vi "Update tsettings from default_Core.vi"(6 "cRIO System Settings Cluster IN 2":T1={"CONFIG Folder - Relative Path "=path "Config", "FIFO Depth (# of elements)"=500000, "Avoid ALARM/ TRIP in transient regimes?"=TRUE, "Sample Rate [Hz]"=2048.0, "Processing interval [s]"=1.0, "Total number of channels to read from FPGA  (auto-calculated)"=0, "# of data to read-DMA (auto-calculated)"=0, "SysLog Interval (s)"=1, "Running Log Folder - Relative Path "=path "Logs/Running_Log", "Reset Log File - Relative Path "=path "Logs/ResetLog/cRIO_reset.txt", "Error Log File - Relative Path "=path "Logs/ErrLog/Errlogs.txt", "Ring Buffer Size (# Log File Elements)"=86400, "CPU Usage Exceed Limit ()"=98.0, "CPU Usage Exceed Limit Delay (# of iterrations)"=60, "Free Memory Min Avail.  (%)"=15.0, "Base CoDiS Folder"=path "c/CoDiS", "Archive Log Folder - Relative Path "=path "Logs/Archive_Logs", "Avail. Drive Space Limit to do Archive (%)"=20.0, "Mediator IP address"="10.50.10.2", "Mediator Communication TCP/IP Port"=2059, "Used channels (from FPGA) per units -Auto calculated"=[], "# DMA FIFO Fulls File - Relative Path "=path "Logs/ResetLog/Number of DMA FIFO Fulls.txt", "Log Status Parameters in cRIO Ring Buffer"=TRUE, "Channels Input Configuration (has to be defined for all available AI)"=[], "Index to check OL and SC (from FPGA) per units and channels -Auto calculated)"=[], "System not OK? (Auto-calculated)"=FALSE, "System not OK Relay Number (-1 = none, 0,..., MAX)"=-1, "Use normal (T) or inverse (F) relay logic for given relay (size of array equals to number of relays)?"=[], "U32 Relay Output (Auto-calculated)"=0, "cRIO Source"=enum."Not Used", "Check DMA FIFO Full?"=FALSE, "Modbus Settings"={"Modbus Communication Port"=502, "Run as Modbus Server/Slave? (FALSE=Modbus Client/Master)"=TRUE, "Modbus Slave Remote IP Address (if Run as Modbus Server/Slave?=FALSE)"=""}, "Time Synchronization Settings"={"Enable Time Synchronization"=FALSE, "Time Server IP Address (if Enable Time Synchronization=TRUE)"=""}} {"Channels Input Configuration (has to be defined for all available AI)" items=["AC Coupled", "DC Coupled", "IEPE AC Coupled", "Not DSA Channel"]}, 8 "cRIO System Settings Cluster IN":T1={"CONFIG Folder - Relative Path "=path "Config", "FIFO Depth (# of elements)"=500000, "Avoid ALARM/ TRIP in transient regimes?"=TRUE, "Sample Rate [Hz]"=2048.0, "Processing interval [s]"=1.0, "Total number of channels to read from FPGA  (auto-calculated)"=0, "# of data to read-DMA (auto-calculated)"=0, "SysLog Interval (s)"=1, "Running Log Folder - Relative Path "=path "Logs/Running_Log", "Reset Log File - Relative Path "=path "Logs/ResetLog/cRIO_reset.txt", "Error Log File - Relative Path "=path "Logs/ErrLog/Errlogs.txt", "Ring Buffer Size (# Log File Elements)"=86400, "CPU Usage Exceed Limit ()"=98.0, "CPU Usage Exceed Limit Delay (# of iterrations)"=60, "Free Memory Min Avail.  (%)"=15.0, "Base CoDiS Folder"=path "c/CoDiS", "Archive Log Folder - Relative Path "=path "Logs/Archive_Logs", "Avail. Drive Space Limit to do Archive (%)"=20.0, "Mediator IP address"="10.50.10.2", "Mediator Communication TCP/IP Port"=2059, "Used channels (from FPGA) per units -Auto calculated"=[], "# DMA FIFO Fulls File - Relative Path "=path "Logs/ResetLog/Number of DMA FIFO Fulls.txt", "Log Status Parameters in cRIO Ring Buffer"=TRUE, "Channels Input Configuration (has to be defined for all available AI)"=[3, 3, 3, 3, 3, 3, 3, 3, 3, 3, 3, 3, 3, 3, 3, 3, 3, 3, 3, 3, 3, 3, 3, 3, 3, 3, 3, 3, 3, 3, 3, 3, 3, 3, 3, 3, 3, 3, 3, 3, 3, 3, 3, 3, 3, 3, 3, 3, 2, 2, 2, 2, 2, 2, 2, 2, 2, 2, 2, 2], "Index to check OL and SC (from FPGA) per units and channels -Auto calculated)"=[], "System not OK? (Auto-calculated)"=FALSE, "System not OK Relay Number (-1 = none, 0,..., MAX)"=-1, "Use normal (T) or inverse (F) relay logic for given relay (size of array equals to number of relays)?"=[TRUE, TRUE, TRUE, TRUE, TRUE, TRUE, TRUE, TRUE], "U32 Relay Output (Auto-calculated)"=0, "cRIO Source"=enum."Source 1", "Check DMA FIFO Full?"=FALSE, "Modbus Settings"={"Modbus Communication Port"=502, "Run as Modbus Server/Slave? (FALSE=Modbus Client/Master)"=TRUE, "Modbus Slave Remote IP Address (if Run as Modbus Server/Slave?=FALSE)"=""}, "Time Synchronization Settings"={"Enable Time Synchronization"=FALSE, "Time Server IP Address (if Enable Time Synchronization=TRUE)"=""}} {"Channels Input Configuration (has to be defined for all available AI)" items=["AC Coupled", "DC Coupled", "IEPE AC Coupled", "Not DSA Channel"]}, 9 "1D array of Pan Cluster IN":T12[](array[typedef]) {"Absolute Minimum Air Gap per Plane"."Absolute AG Minimum Pole Number" format="%.3f"; "Absolute Minimum Air Gap per Plane"."Absolute AG Minimum Value" format="%.3f"; "Magnetic Field Data"."Maximum by Pole Number" format="%.3f"; "Air Gap Data"."Minimum by Pole Number" format="%.3f"; "Orbit(s) - XY"."Orbit XY Graphs (Synthesized from Selected Harmonics and DC)"."?" format="%.3f"; "Orbit(s) - XY"."Orbit XY Graphs (Synthesized from Selected Harmonics and DC)"."?" format="%.3f"; "Orbit(s) - XY"."Orbit XY Graphs (Glided and Averaged on One Revolution)"."?" format="%.3f"; "Orbit(s) - XY"."Orbit XY Graphs (Glided and Averaged on One Revolution)"."?" format="%.3f"; "Orbit(s) - XY"."Orbit XY Graphs (Unaveraged)"."?" format="%.3f"; "Orbit(s) - XY"."Orbit XY Graphs (Unaveraged)"."?" format="%.3f"}, 10 "1D array of Waveform Cluster IN":T6[](array[typedef]) {"Analysis Parameters"."SP2Pmax"."Filter Parameters"."low cutoff freq: fl" format="%0.4f"; "Analysis Parameters"."SP2Pmax"."Filter Parameters"."high cutoff freq: fh" format="%0.2f"; "Analysis Parameters"."LoadAngleDelta"."Multiplication Factor" format="%.1f"; "Analysis Parameters"."LoadAngleDelta"."What harmonic? (for example 24th (48 pole machine))" format="%.1f"; "Analysis Parameters"."Peak2Peak"."Filter Parameters"."low cutoff freq: fl" format="%0.4f"; "Analysis Parameters"."Peak2Peak"."Filter Parameters"."high cutoff freq: fh" format="%0.2f"; "Analysis Parameters"."RMS"."Filter Parameters"."order" format="%0.4f"; "Analysis Parameters"."RMS"."Filter Parameters"."low cutoff freq: fl" format="%0.2f"; "Analysis Parameters"."RMS"."Filter Parameters"."high cutoff freq: fh" format="%0.2f"; "Analysis Parameters"."EqPeak"."Filter Parameters"."low cutoff freq: fl" format="%0.4f"; "Analysis Parameters"."EqPeak"."Filter Parameters"."high cutoff freq: fh" format="%0.2f"; "Analysis Parameters"."Peak"."Filter Parameters"."low cutoff freq: fl" format="%0.4f"; "Analysis Parameters"."Peak"."Filter Parameters"."high cutoff freq: fh" format="%0.2f"; "Analysis Parameters"."snPh"."What harmonic?" format="%.1f"; "Analysis Parameters"."snA"."Multiplication Factor" format="%.1f"; "Analysis Parameters"."snA"."What harmonic?" format="%.1f"; "Analysis Parameters"."Smax"."Filter Parameters"."low cutoff freq: fl" format="%0.4f"; "Analysis Parameters"."Smax"."Filter Parameters"."high cutoff freq: fh" format="%0.2f"; "Analysis Parameters"."RPM"."Signal Threshold" format="%.1f"}, 11 "System_settings IN":T4={"Units in the system"=[], "dBase names by units"=[], "TCP/IP processing units addresses"=[], "TCP/IP server address"="", "dBase User Name_Cli"="codis_cli", "dBase User Password_Cli"="codis_cli", "dBase User Name_Med"="codis_med_wrt", "dBase User Password_Med"="codis_med_wrt", "Sampling rate [Hz]"=0.0, "FTP Server User name, cRIO"="", "FTP Server Password, cRIO"="", "OnScreenKeyboardPopUp"=FALSE, "Number of points to collect"=0, "Main Window has title bar?"=FALSE, "Demo?"=FALSE, "dBase - Limit # of  elements to read"=0, "dBase Backup"={"dBase Backup Base Folder"="c:\\codis\\backup\\", "Remote dBase Backup Configured?"=TRUE}, "System Status"={"System Monitor Refresh Rate (ms)"=10000, "System Status Log  File"="c:\\codis\\system_info.txt", "Max number of elements to read\n"=26611200}, "Number of points to average for stationary state"=[60], "Number of points to collect for saving waveforms per channel"=[60], "Sources per Unit"=[], "TCP/IP_client_mediator_communication ports"=2058, "TCP/IP processing_units _mediator_communication ports"=2055}) -> ()   [LabVIEW 2014]
uses:
  common/typedefs/Pan_Cluster_Core.ctl
  common/typedefs/Condition_Vector_Cluster_Core.ctl
  common/typedefs/Unit_Names_Core.ctl
  common/typedefs/Data_Sources_Core.ctl
  common/typedefs/Waveforms_Cluster_Core.ctl
  common/typedefs/Types_of_Signals_Core.ctl
  common/typedefs/Types_of_Analyses_Core.ctl
  common/typedefs/Analysis_Parameters_Cluster_Core.ctl
  <vilib>/Analysis/3filter.llb/Filter Passband Type.ctl
  common/typedefs/Integration_Types_Core.ctl
  common/typedefs/System_Settings_Cluster_Client_Mediator_Core.ctl
  common/typedefs/cRIO_System_Settings_Cluster_Core.ctl
  common/typedefs/DSA_Channels_Configuration_Core.ctl
  common/typedefs/dBase_Tables_Core.ctl
  common/typedefs/tsettings_Core.ctl
  <vilib>/addons/database/Connection.llb/DB Tools Open Connec (String).vi
  <vilib>/addons/database/NI_Database_API.lvlib
  <vilib>/Analysis/NI_AALBase.lvlib
panel:
  out "error out":errorcluster
  out "file error":errorcluster
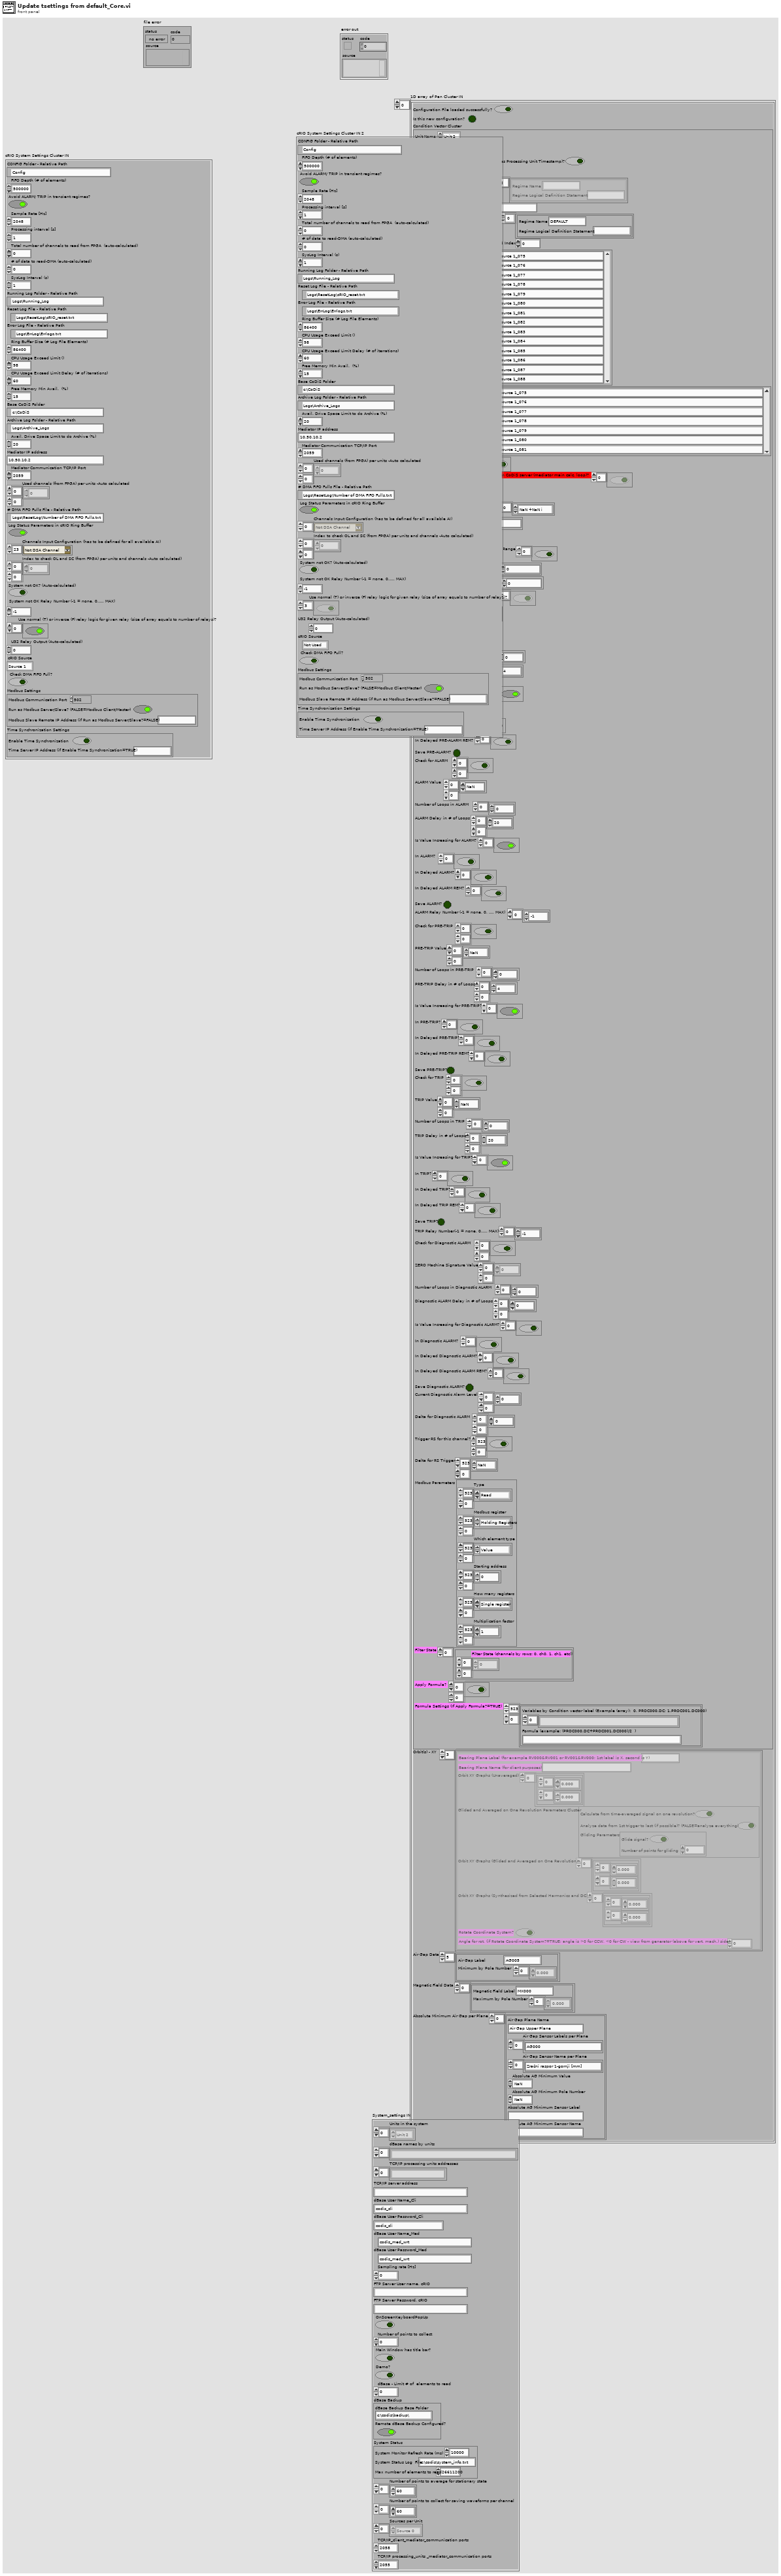
[diagram p1: front panel]
types:
  T1 = typedef "cRIO_System_Settings_Cluster_Core.ctl" = cluster{"CONFIG Folder - Relative Path ":path, "FIFO Depth (# of elements)":u32, "Avoid ALARM/ TRIP in transient regimes?":bool, "Sample Rate [Hz]":sgl, "Processing interval [s]":sgl, "Total number of channels to read from FPGA  (auto-calculated)":u32, "# of data to read-DMA (auto-calculated)":u32, "SysLog Interval (s)":u32, "Running Log Folder - Relative Path ":path, "Reset Log File - Relative Path ":path, "Error Log File - Relative Path ":path, "Ring Buffer Size (# Log File Elements)":u32, "CPU Usage Exceed Limit ()":sgl, "CPU Usage Exceed Limit Delay (# of iterrations)":u32, "Free Memory Min Avail.  (%)":sgl, "Base CoDiS Folder":path, "Archive Log Folder - Relative Path ":path, "Avail. Drive Space Limit to do Archive (%)":sgl, "Mediator IP address":string, "Mediator Communication TCP/IP Port":u16, "Used channels (from FPGA) per units -Auto calculated":i32[][], "# DMA FIFO Fulls File - Relative Path ":path, "Log Status Parameters in cRIO Ring Buffer":bool, "Channels Input Configuration (has to be defined for all available AI)":T2[], "Index to check OL and SC (from FPGA) per units and channels -Auto calculated)":i32[][], "System not OK? (Auto-calculated)":bool, "System not OK Relay Number (-1 = none, 0,..., MAX)":i16, "Use normal (T) or inverse (F) relay logic for given relay (size of array equals to number of relays)?":bool[], "U32 Relay Output (Auto-calculated)":u32, "cRIO Source":T3, "Check DMA FIFO Full?":bool, "Modbus Settings":cluster{"Modbus Communication Port":u16, "Run as Modbus Server/Slave? (FALSE=Modbus Client/Master)":bool, "Modbus Slave Remote IP Address (if Run as Modbus Server/Slave?=FALSE)":string}, "Time Synchronization Settings":cluster{"Enable Time Synchronization":bool, "Time Server IP Address (if Enable Time Synchronization=TRUE)":string}}
  T2 = typedef "DSA_Channels_Configuration_Core.ctl" = u16
  T3 = typedef "Data_Sources_Core.ctl" = enum16{"Not Used", "Source 0", "Source 1", "Source 2", "Source 3", "Source 4", "Source 5", "Source 6", "Source 7", "Source 8", "Source 9", "Source 10", "Source 11", "Source 12", "Source 13", "Source 14", "Source 15", "Source 16", "Source 17", "Source 18", "Source 19", "Source 20"}
  T4 = typedef "System_Settings_Cluster_Client_Mediator_Core.ctl" = cluster{"Units in the system":T5[], "dBase names by units":string[], "TCP/IP processing units addresses":string[], "TCP/IP server address":string, "dBase User Name_Cli":string, "dBase User Password_Cli":string, "dBase User Name_Med":string, "dBase User Password_Med":string, "Sampling rate [Hz]":dbl, "FTP Server User name, cRIO":string, "FTP Server Password, cRIO":string, "OnScreenKeyboardPopUp":bool, "Number of points to collect":u32, "Main Window has title bar?":bool, "Demo?":bool, "dBase - Limit # of  elements to read":u32, "dBase Backup":cluster{"dBase Backup Base Folder":string, "Remote dBase Backup Configured?":bool}, "System Status":cluster{"System Monitor Refresh Rate (ms)":u32, "System Status Log  File":string, "Max number of elements to read\n":i64}, "Number of points to average for stationary state":i32[], "Number of points to collect for saving waveforms per channel":i32[], "Sources per Unit":T3[], "TCP/IP_client_mediator_communication ports":u16, "TCP/IP processing_units _mediator_communication ports":u16}
  T5 = typedef "Unit_Names_Core.ctl" = enum16{"Not used", "Unit 1", "Unit 2", "Unit 3", "Unit 4", "Unit 5", "Unit 6", "Unit 7", "Unit 8", "Unit 9"}
  T6 = typedef "Waveforms_Cluster_Core.ctl" = cluster{"Configuration File loaded successfully? ":bool, "Is this new configuration?":bool, "Unit Name":T5, "Waveform Source":T3[], "Use CoDiS server Timestamp (on FALSE uses Processing Unit Timestamp)?":bool, "Sampling Rate [Hz]":u32[], "Timestamp (DBL)":dbl, "Mode of Operation - Normal":string, "Mode of Operation - Diagnostic":string, "Waveform Physical Channel":u16[], "Waveform Label":string[], "Waveform Name":string[], "Signal Type":cluster{"Signal Type":T7, "# of signal of particular type":u8}[], "Is this Main Trigger Signal?":bool[], "Slope":dbl[], "Intercept":dbl[], "Waveform Values":sgl[][], "Analyse?":bool[], "Save to database?":bool[], "Analyses to Perform":T8[][], "Perform this analysis on a CoDiS server?":bool[][], "General Parameters":cluster{"Number of Poles":u8, "Grid Frequency":sgl}, "Analysis Parameters":T9[][], "Save now to dBase?":bool, "Waveform Length for Saving [s]":u16, "Pretrigger Length when Saving Waveform [s]":u16, "Next Timestamp to autosave at (DBL)":dbl, "Description of Waveforms Events":string, "Event Type":string, "Save next RS event entirely? (on FALSE uses How many basic (acquisition) blocks of data (loops) to save?":bool, "Regime Name for which to save next RS event entirely":string, "Integration type":T11[], "Channel not OK?":bool[], "Channel Not OK?  Relay Number (-1 = none, 0, ..., MAX)":i16[], "Array of FPGA Filter Parameters":cluster{"Filter signal?":bool, "filter type":T10, "high cutoff freq: fh":dbl, "low cutoff freq: fl":dbl, "order":i32}[][], "Pre-Alarm Delay in Number of Loops ":u16, "Pre-Trip Delay in Number of Loops ":u16}
  T7 = typedef "Types_of_Signals_Core.ctl" = enum16{"Not Used", "Trigger (TRG???)", "Relative Vibrations (RV???)", "Absolute Vibrations (AV???)", "Air Gap (AG???)", "Magnetic Field (MX???)", "Voltage (VOL???)", "Current (CURR???)", "Process (PROC???)", "Cavitation (CAV???)", "Non Standard (NONST???)", "Axial Displacement (AXD???)", "Absolute Vibrations Stator Core (AVSC???)"}
  T8 = typedef "Types_of_Analyses_Core.ctl" = enum16{"Exit Analysis Loop", "Do Nothing", "RPM", "Smax", "SP2Pmax", "snA", "snPh", "Rest", "Peak", "EqPeak", "Peak2Peak", "RMS", "DC", "DC from Extrema", "Min Value", "Max Value", "Min Value by Pole", "Max Value by Pole", "Max Diff by Pole", "Max Diff Pole Number", "Min from Extrema", "Max from Extrema", "Active Power from DFT", "Active Power by Integration", "Reactive Power from DFT", "Reactive Power by Integration", "Apparent Power", "Ampl@Freq", "Phase Difference", "Load Angle Delta", "THD", "Signal Frequency", "Eta", "Non standard (CoDiS server - manual) 0", "Non standard (CoDiS server - manual) 1", "Non standard (CoDiS server - manual) 2", "Non standard (CoDiS server - manual) 3", "Non standard (CoDiS server - manual) 4", "Non standard (CoDiS server - manual) 5", "Non standard (CoDiS server - manual) 6", "Non standard (CoDiS server - manual) 7", "Non standard (CoDiS server - manual) 8", "Non standard (CoDiS server - manual) 9", "Non standard (CoDiS server - manual) 10", "Non standard (CoDiS server - manual) 11", "Non standard (CoDiS server - manual) 12", "Non standard (CoDiS server - manual) 13", "Non standard (CoDiS server - manual) 14", "Non standard (CoDiS server - manual) 15", "Non standard (CoDiS server - manual) 16", "Non standard (CoDiS server - manual) 17", "Non standard (CoDiS server - manual) 18", "Non standard (CoDiS server - manual) 19", "CosFi", "Total THD", "Crest Factor"}
  T9 = typedef "Analysis_Parameters_Cluster_Core.ctl" = cluster{"DC":cluster{"Analyze data from 1st trigger to last (if possible)? (FALSE=analyze everything)":bool}, "DCExtrema":cluster{"Calculate DC from all Pole Values":bool, "Poles to use in DC calculation (if Calculate DC from all Pole Values is FALSE)":u8[], "Condition Vector Label begin Part (MinPole or MaxPole)":string, "Addition to Condition Vector Label (example: 000)":string}, "RPM":cluster{"Signal Threshold":sgl, "Pulse Width (should be >= 2 depending on signal noise)":i32, "Trigger on rising edge? (FALSE=trigger on falling)":bool}, "Smax":cluster{"Combine with which Waveform Label? (for example: RV001)":string, "Calculate from time-averaged signal on one revolution?":bool, "Analyze data from 1st trigger to last (if possible)? (FALSE=analyze everything)":bool, "Filter Parameters":cluster{"Filter signal?":bool, "filter type":T10, "high cutoff freq: fh":dbl, "low cutoff freq: fl":dbl, "order":i32, "Process as ring-buffer signal?":bool}, "Gliding Parameters":cluster{"Glide signal?":bool, "Number of points for gliding":u16}, "Average all calculated values for Smax - if present (each revolution)? (FALSE=take absolute maximum)":bool, "Addition to Condition Vector Label (example: 000)":string}, "SP2Pmax":cluster{"Combine with which Waveform Label? (for example: RV001)":string, "Calculate from time-averaged signal on one revolution?":bool, "Analyze data from 1st trigger to last (if possible)? (FALSE=analyze everything)":bool, "Filter Parameters":cluster{"Filter signal?":bool, "filter type":T10, "high cutoff freq: fh":dbl, "low cutoff freq: fl":dbl, "order":i32, "Process as ring-buffer signal?":bool}, "Gliding Parameters":cluster{"Glide signal?":bool, "Number of points for gliding":u16}, "Average all calculated values for SP2Pmax - if present (each revolution)? (FALSE=take absolute maximum)":bool, "Addition to Condition Vector Label (example: 000)":string}, "snA":cluster{"What harmonic?":sgl, "Calculate Amplitude (TRUE) or RMS (FALSE)?":bool, "Multiplication Factor":sgl, "Calculate Amplitude for Air Gap type signals? (from MinPole Values)":bool}, "snPh":cluster{"What harmonic?":sgl}, "Peak":cluster{"Calculate from time-averaged signal (one-revolution)?":bool, "Analyze data from 1st trigger to last (if possible)? (FALSE=analyze everything)":bool, "Filter Parameters":cluster{"Filter signal?":bool, "filter type":T10, "high cutoff freq: fh":dbl, "low cutoff freq: fl":dbl, "order":i32, "Process as ring-buffer signal?":bool}, "Gliding Parameters":cluster{"Glide signal?":bool, "Number of points for gliding":u16}, "Average all calculated values for Peak - if present (each revolution)? (FALSE=take absolute maximum)":bool, "Addition to Condition Vector Label (example: 000)":string}, "Peak2Peak":cluster{"Calculate from time-averaged signal (one-revolution)?":bool, "Analyze data from 1st trigger to last (if possible)? (FALSE=analyze everything)":bool, "Gliding Parameters":cluster{"Glide signal?":bool, "Number of points for gliding":u16}, "Filter Parameters":cluster{"Filter signal?":bool, "filter type":T10, "high cutoff freq: fh":dbl, "low cutoff freq: fl":dbl, "order":i32, "Process as ring-buffer signal?":bool}, "Average all calculated values for Peak2Peak - if present (each revolution)? (FALSE=take absolute maximum)":bool, "Addition to Condition Vector Label (example: 000)":string}, "EqPeak":cluster{"Calculate from time-averaged signal (one-revolution)?":bool, "Analyze data from 1st trigger to last (if possible)? (FALSE=analyze everything)":bool, "Average all calculated values for EqPeak - if present (each revolution)? (FALSE=take absolute maximum)":bool, "Filter Parameters":cluster{"Filter signal?":bool, "filter type":T10, "high cutoff freq: fh":dbl, "low cutoff freq: fl":dbl, "order":i32, "Process as ring-buffer signal?":bool}, "Which Condition Vector Label addition to use for RMS (example: 001)":string, "Addition to Condition Vector Label (example: 000)":string}, "RMS":cluster{"Calculate from time-averaged signal (one-revolution)?":bool, "Analyze data from 1st trigger to last (if possible)? (FALSE=analyze everything)":bool, "Subtract DC before RMS calculation?":bool, "Filter Parameters":cluster{"Filter signal?":bool, "filter type":T10, "high cutoff freq: fh":dbl, "low cutoff freq: fl":dbl, "order":i32, "Process as ring-buffer signal?":bool}, "Gliding Parameters":cluster{"Glide signal?":bool, "Number of points for gliding":u16}, "Average all calculated values for RMS - if present (each revolution)? (FALSE=take absolute maximum)":bool, "Addition to Condition Vector Label (example: 000)":string}, "Rest":cluster{"Calculate from all calculated harmonics?":bool, "Condition Vector Label to use for substraction (if Calculate from all calculated harmonics?=FALSE)":string[], "Calculate by subtracting from EqPeak Value? (FALSE=calculate by subtracting from RMS Value)":bool, "Which Condition Vector Label addition to use for EqPeak (example: 001)":string, "Addition to Condition Vector Label (example: 000)":string}, "MinByPole":cluster{"First Pole Number after Trigger (indexes correspond to Normal regime settings)":u8[], "Are Pole Numbers in ascending order in time?  (indexes correspond to Normal regime settings)":bool[], "Average all calculated values for that Pole? (FALSE=take absolute minimum)":bool, "Coerce Upper Limit":sgl, "Compensate 1st harmonic in waveform?":bool}, "MinExtrema":cluster{"Calculate Min Extrema from all Pole Values":bool, "Poles to use in Min Extrema calculation (if Calculate Min Extrema from all Pole Values is FALSE)":u8[], "Condition Vector Label begin Part (MinPole or MaxPole)":string}, "MaxByPole":cluster{"First Pole Number after Trigger (indexes correspond to Normal regime settings)":u8[], "Are Pole Numbers in ascending order in time? (indexes correspond to Normal regime settings)":bool[], "Average all calculated values for that Pole? (FALSE=take absolute maximum)":bool, "Calculate with abs(Signal)?":bool, "Subtract DC before calculation?":bool, "Coerce Lower Limit":sgl}, "MaxExtrema":cluster{"Calculate Max Extrema from all Pole Values":bool, "Poles to use in Max Extrema calculation (if Calculate Max Extrema from all Pole Values is FALSE)":u8[], "Condition Vector Label begin Part (MinPole or MaxPole)":string}, "MaxDiffByPole":cluster{"First Pole Number after Trigger (indexes correspond to Normal regime settings)":u8[], "Are Pole Numbers in ascending order in time? (indexes correspond to Normal regime settings)":bool[], "Condition Vector Label begin Part (MinPole or MaxPole)":string}, "Min":cluster{"Analyze data from 1st trigger to last (if possible)? (FALSE=analyze everything)":bool, "Calculate from time-averaged signal on one revolution?":bool, "Gliding Parameters":cluster{"Glide signal?":bool, "Number of points for gliding":u16}, "Average all calculated values for Min - if present (each revolution)? (FALSE=take absolute maximum)":bool}, "Max":cluster{"Analyze data from 1st trigger to last (if possible)? (FALSE=analyze everything)":bool, "Calculate from time-averaged signal on one revolution?":bool, "Gliding Parameters":cluster{"Glide signal?":bool, "Number of points for gliding":u16}, "Average all calculated values for Max - if present (each revolution)? (FALSE=take absolute maximum)":bool}, "ActivePower":cluster{"Calculate from Phase Voltages and Currents?":bool, "Phase Voltage Condition Vector Label (R, S, T) (for example: VOL000.s24.00A, VOL001.s24.00A, VOL002.s24.00A)":string[], "Phase Current Condition Vector Label (R, S, T) (for example: CURR000.s24.00A, CURR001.s24.00A, CURR002.s24.00A)":string[]}, "ReactivePower":cluster{"Calculate from Phase Voltages and Currents?":bool, "Phase Voltage Condition Vector Label (R, S, T) (for example: VOL000.s24.00A, VOL001.s24.00A, VOL002.s24.00A)":string[], "Phase Current Condition Vector Label (R, S, T) (for example: CURR000.s24.00A, CURR001.s24.00A, CURR002.s24.00A)":string[]}, "LoadAngleDelta":cluster{"What harmonic? (for example 24th (48 pole machine))":sgl, "Delta0":sgl, "Which Voltage Waveform Label? (for example: VOL000)":string, "Combine (multiply) with which Air Gap Waveform Label? (for example: AG000)":string, "Multiplication Factor":sgl}, "ActivePowerByIntegration":cluster{"Phase Voltage Waveform Labels (R,S,T)":string[], "Phase Current Waveform Labels (R,S,T)":string[], "Analyze data from 1st trigger to last (if possible)? (FALSE=analyze everything)":bool}, "RectivePowerByIntegration":cluster{"Phase Voltage Waveform Vector Labels (R,S,T)":string[], "Phase Current Waveform Labels (R,S,T)":string[], "System Electric Frequency [Hz]":sgl, "Analyze data from 1st trigger to last (if possible)? (FALSE=analyze everything)":bool}, "Ampl@Freq":cluster{"Frequency [Hz]":sgl, "Calculate Amplitude? (FALSE=calculate RMS)":bool}, "PhaseDifference":cluster{"Combine with which Waveform Label?":string}, "CosFi":cluster{"Voltage Waveform Labels (R,S,T)":string[], "Current Waveform Labels (R,S,T)":string[]}, "Total THD":cluster{"THD Condition Vector Label (R, S, T) (for example: VOL000.THD, VOL001.THD, VOL002.THD)":string[]}, "Crest Factor":cluster{"Addition to Condition Vector Label (example: 000)":string, "Which Condition Vector Label addition to use for Peak (example: 001)":string, "Which Condition Vector Label addition to use for RMS (example: 001)":string}}
  T10 = typedef "NI_AALBase.lvlib/Filter Passband Type.ctl" = enum32{"Lowpass", "Highpass", "Bandpass", "Bandstop"}
  T11 = typedef "Integration_Types_Core.ctl" = enum16{"Do not integrate", "Integrate once", "Integrate twice"}
  T12 = typedef "Pan_Cluster_Core.ctl" = cluster{"Configuration File loaded successfully?":bool, "Is this new configuration?":bool, "Condition Vector Cluster":T13, "Orbit(s) - XY":cluster{"Bearing Plane Label (for example RV000&RV001 or RV001&RV000; 1st label is X, second is Y)":string, "Bearing Plane Name (for client purposes)":string, "Orbit XY Graphs (Unaveraged)":cluster{sgl[], sgl[]}[], "Glided and Averaged on One Revolution Parameters Cluster":cluster{"Calculate from time-averaged signal on one revolution?":bool, "Analyze data from 1st trigger to last (if possible)? (FALSE=analyze everything)":bool, "Gliding Parameters":cluster{"Glide signal?":bool, "Number of points for gliding":u16}}, "Orbit XY Graphs (Glided and Averaged on One Revolution)":cluster{sgl[], sgl[]}[], "Orbit XY Graphs (Synthesized from Selected Harmonics and DC)":cluster{sgl[], sgl[]}[], "Rotate Coordinate System?":bool, "Angle for rot. (if Rotate Coordinate System?=TRUE; angle is >0 for CCW, <0 for CW - view from generator (above for vert. mach.) side)":sgl}[], "Air Gap Data":cluster{"Air Gap Label":string, "Minimum by Pole Number":sgl[]}[], "Magnetic Field Data":cluster{"Magnetic Field Label":string, "Maximum by Pole Number":sgl[]}[], "Absolute Minimum Air Gap per Plane":cluster{"Air Gap Plane Name":string, "Air Gap Sensor Labels per Plane":string[], "Air Gap Sensor Name per Plane":string[], "Absolute AG Minimum Value":sgl, "Absolute AG Minimum Pole Number":sgl, "Absolute AG Minimum Sensor Label":string, "Absolute AG Minimum Sensor Name":string}[]}
  T13 = typedef "Condition_Vector_Cluster_Core.ctl" = cluster{"Unit Name":T5, "Source Name":T3[], "Use CoDiS server Timestamp (on FALSE uses Processing Unit Timestamp)?":bool, "Timestamp (DBL)":dbl, "Mode of Operation - Normal (Settings)":cluster{"Regime Name":string, "Regime Logical Definition Statement":string}[], "Mode of Operation - Normal":string, "Mode of Operation - Diagnostic (Settings)":cluster{"Regime Name":string, "Regime Logical Definition Statement":string}[], "Mode of Operation - Diagnostic Recognized Index":i16, "Condition Vector Label":string[], "Condition Vector Name":string[], "Is this Main Trigger Signal?":bool[], "Perform PRE-ALARM, ALARM, etc. Analysis on CoDiS server (mediator main calc. loop)?":bool[], "Trigger Indexes":u32[], "Condition Vector Values Complex (CDB)":cdb[], "Condition Vector Values":sgl[], "Save to dBase":bool[], "Check if Condition Vector Element is out of Range":bool[], "Condition Vector Low Limit Value":sgl[], "Condition Vector High Limit Value":sgl[], "Condition Vector Element out of Range":bool[], "Check for PRE-ALARM":bool[][], "PRE-ALARM Value":sgl[][], "Number of Loops in PRE-ALARM":u32[], "PRE-ALARM Delay in # of Loops":u16[][], "Is Value Increasing for PRE-ALARM?":bool[], "In PRE-ALARM?":bool[], "In Delayed PRE-ALARM?":bool[], "In Delayed PRE-ALARM REM?":bool[], "Save PRE-ALARM?":bool, "Check for ALARM":bool[][], "ALARM Value":sgl[][], "Number of Loops in ALARM":u32[], "ALARM Delay in # of Loops":u16[][], "Is Value Increasing for ALARM?":bool[], "In ALARM?":bool[], "In Delayed ALARM?":bool[], "In Delayed ALARM REM?":bool[], "Save ALARM?":bool, "ALARM Relay Number (-1 = none, 0, ..., MAX)":i16[], "Check for PRE-TRIP":bool[][], "PRE-TRIP Value":sgl[][], "Number of Loops in PRE-TRIP":u32[], "PRE-TRIP Delay in # of Loops":u16[][], "Is Value Increasing for PRE-TRIP?":bool[], "In PRE-TRIP?":bool[], "In Delayed PRE-TRIP?":bool[], "In Delayed PRE-TRIP REM?":bool[], "Save PRE-TRIP?":bool, "Check for TRIP":bool[][], "TRIP Value":sgl[][], "Number of Loops in TRIP":u32[], "TRIP Delay in # of Loops":u16[][], "Is Value Increasing for TRIP?":bool[], "In TRIP?":bool[], "In Delayed TRIP?":bool[], "In Delayed TRIP REM?":bool[], "Save TRIP?":bool, "TRIP Relay Number(-1 = none, 0,..., MAX)":i16[], "Check for Diagnostic ALARM":bool[][], "ZERO Machine Signature Value":dbl[][], "Number of Loops in Diagnostic ALARM":u32[], "Diagnostic ALARM Delay in # of Loops":u16[][], "Is Value Increasing for Diagnostic ALARM?":bool[], "In Diagnostic ALARM?":bool[], "In Delayed Diagnostic ALARM?":bool[], "In Delayed Diagnostic ALARM REM?":bool[], "Save Diagnostic ALARM?":bool, "Current Diagnostic Alarm Level":sgl[][], "Delta for Diagnostic ALARM":sgl[][], "Trigger RS for this channel?":bool[][], "Delta for RS Trigger":sgl[][], "Modbus Parameters":cluster{"Type":enum16{"Read", "Write", "None"}[][], "Modbus register":enum16{"Coils", "Discrete Inputs", "Input Registers", "Holding Registers"}[][], "Which element type":enum16{"Value", "Alarm", "Trip"}[][], "Starting address":u16[][], "How many registers":enum16{"Single register", "HI-LO", "LO-HI"}[][], "Multiplication factor":dbl[][]}, "Filter State":cluster{"Filter State (channels by rows: 0. ch0, 1. ch1, etc))":dbl[][]}[], "Apply Formula?":bool[][], "Formula Settings (If Apply Formula?=TRUE)":cluster{"Variables by Condition vector label (Example (array):  0. PROC000.DC; 1.PROC001.DC000)":string[], "Formula (example: (PROC000.DC+PROC001.DC000)/2  )":string}[][]}
  T14 = typedef "tsettings_Core.ctl" = enum16{"Waveform Cluster", "Pan Cluster", "Reference Waveform for AG RSS", "System Settings", "RunOut Vector"}
  T15 = typedef "dBase_Tables_Core.ctl" = string
  T16 = typedef "NI_Database_API.lvlib/Conn ObjectReference.ctl" = refnum<k1>
  T17 = cluster{"Number of records OUT":u64, "idUser":u64, "tSetting_TypeDef":T14, dbl, "Waveform Cluster DEFAULT":T6, "Administrator Cluster.Description":string, "Uploaded":u64}
  T18 = cluster{u64, "idUser":u64, i32, dbl, "cRIO System Settings Cluster IN 2":T1, "Administrator Cluster.Description":string, "Uploaded":u64}
  T19 = cluster{u64, "idUser":u64, "tSetting_TypeDef":T14, dbl, "Pan Cluster DEFAULT":T12, "Administrator Cluster.Description":string, "Uploaded":u64}
  T20 = cluster{u64, "idUser":u64, i32, dbl, "cRIO System Settings Cluster IN":T1, "Administrator Cluster.Description":string, "Uploaded":u64}
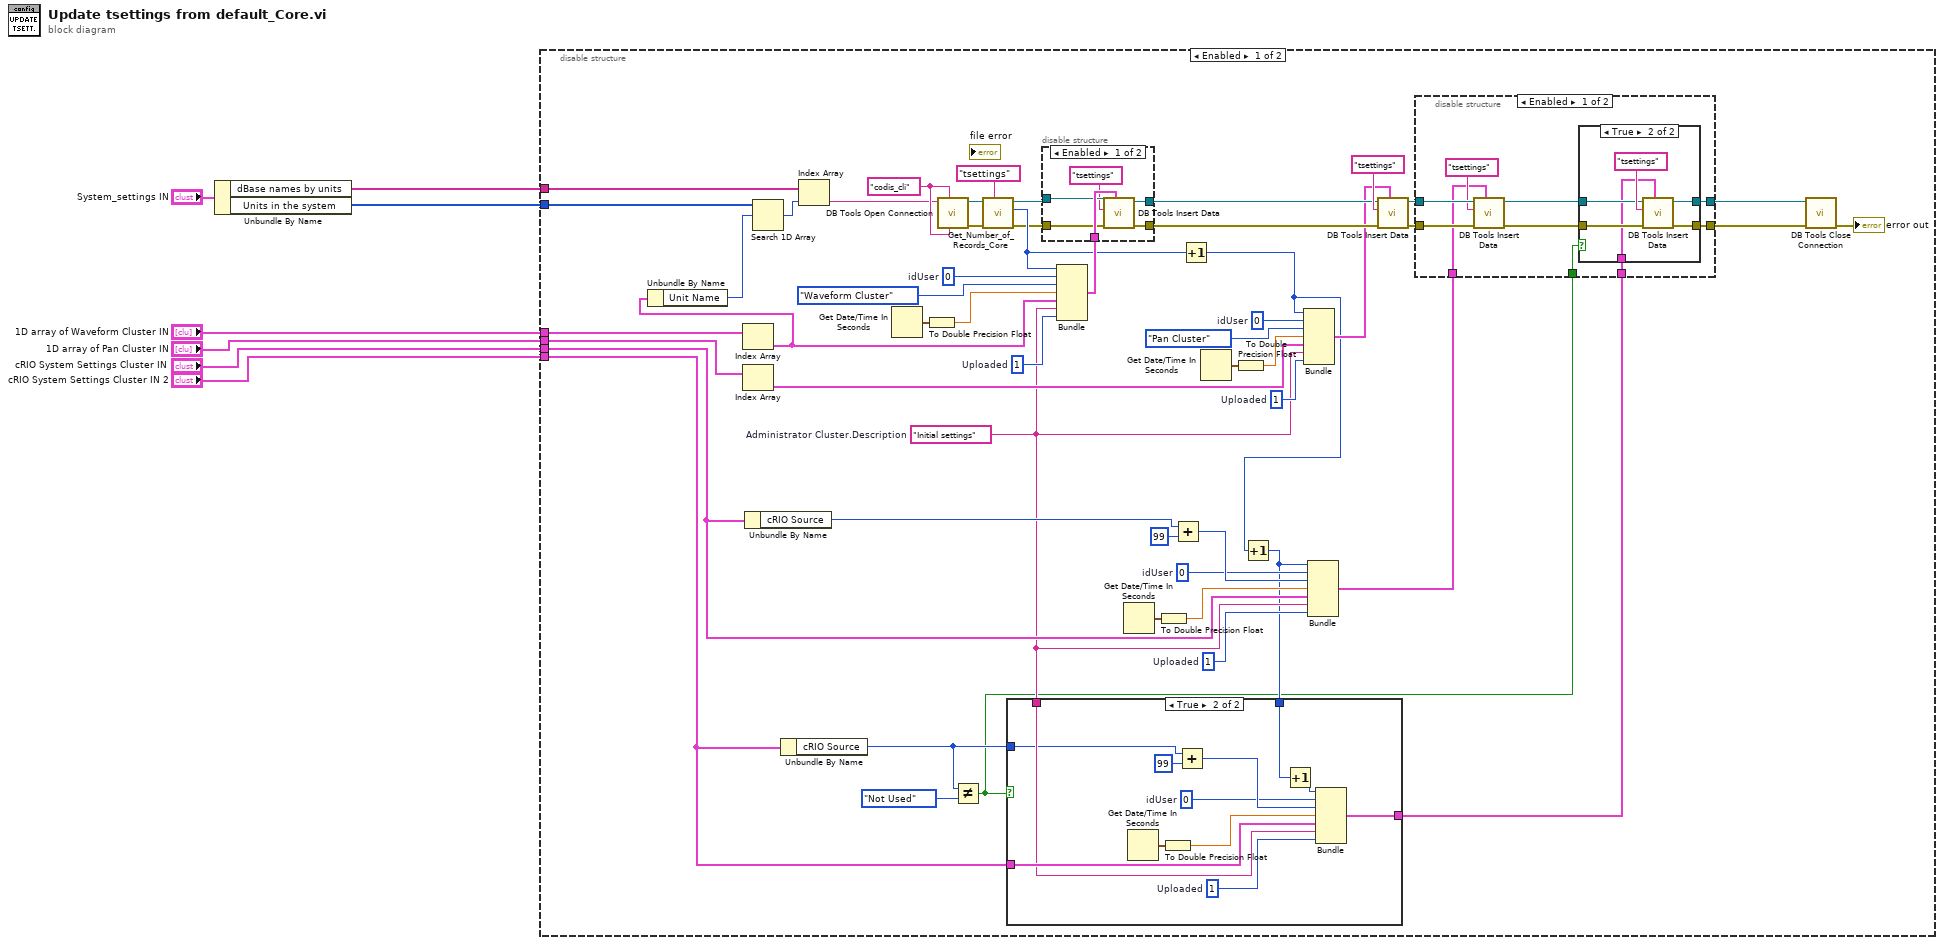
[diagram p0: block diagram]
diagram:
  n1 = Unbundle By Name("System_settings IN") -> ("dBase names by units"=w6:string[], "Units in the system"=w7:T5[])
  n2 = disable-structure shown="Enabled" {
    disable-tunnel: "1D array of Waveform Cluster IN" -> [w44 _]
    disable-tunnel: "1D array of Pan Cluster IN" -> [w43 _]
    disable-tunnel: "cRIO System Settings Cluster IN" -> [w34 _]
    disable-tunnel: "cRIO System Settings Cluster IN 2" -> [w30 _]
    disable-tunnel: w7 -> [w24 _]
    disable-tunnel: w6 -> [w21 _]
    frame Enabled {
      w41 = u64 1  # Uploaded
      w28 = u64 0  # idUser
      w29 = "Initial settings"  # Administrator Cluster.Description
      w52 = u64 1  # Uploaded
      w53 = u64 0  # idUser
      w55 = "codis_cli" ("password")
      w57 = u64 1  # Uploaded
      w58 = u64 0  # idUser
      n3 = Index Array(array=w44) -> (element=w23:T6)  [unwired: 1 in]
      n4 = Unbundle By Name(w23) -> ("Unit Name"=w22:T5)
      n5 = Index Array(array=w43) -> (element=w45:T12)  [unwired: 1 in]
      n6 = Unbundle By Name(w34) -> ("cRIO Source"=w33:T3)
      n7 = Search 1D Array(1D array=w24, element=w22) -> (index of element=w20:i32)  [unwired: 1 in]
      n8 = Unbundle By Name(w30) -> ("cRIO Source"=w17:T3)
      n9 = Index Array(array=w21, index=w20) -> (element=w19:string)
      n10 = Get Date/Time In Seconds() -> (seconds since 1Jan1904=w60:timestamp)
      n11 = To Double Precision Float(number=w60) -> (double precision float=w56:dbl)
      n12 = call-poly <vilib>:"DB Tools Open Connection.vi"("password"=w55, "userID"=w55, "connection information"=w19) -> ("error out"=w14:errorcluster, "connection reference"=w15:T16)  [unwired: 5 in]
      n13 = Not Equal?(x=w17, y=Data_Sources_Core."Not Used" ("cRIO Source")) -> (x != y?=w16:bool)
      n14 = call "Get_Number_of_Records_Core.vi"("Table"=T15 "tsettings", "error IN"=w14, "Connection reference IN"=w15) -> ("error OUT"=w11:errorcluster, "Number of records OUT"=w13:u64, "Connection reference OUT"=w12:T16)  [unwired: 6 in]
      n15 = Bundle("Number of records OUT"=w13, "idUser"=w58, "tSetting_TypeDef"=tsettings_Core."Waveform Cluster", w56, "Waveform Cluster DEFAULT"=w23, "Administrator Cluster.Description"=w29, "Uploaded"=w57) -> (w59:T17)  [unwired: 1 in]
      n16 = disable-structure shown="Enabled" {
        disable-tunnel: w59 -> [w78 _]
        disable-tunnel: w11 -> [w77 w79]
        disable-tunnel: w12 -> [w76 w80]
        disable-tunnel: [w74 w80] -> w49
        disable-tunnel: [w73 w79] -> w48
        frame Enabled {
          n17 = call <vilib>:"DB Tools Insert Data.vi"("data"=w78, "error in (no error)"=w77, "table"="tsettings", "connection reference"=w76) -> ("error out"=w73:errorcluster, "connection reference out"=w74:T16)  [unwired: 6 in]
        }
        frame Disabled {
        }
      }
      n18 = Get Date/Time In Seconds() -> (seconds since 1Jan1904=w40:timestamp)
      n19 = To Double Precision Float(number=w40) -> (double precision float=w42:dbl)
      n20 = Add(x=w33, y=99) -> (x+y=w38:i32)
      n21 = Increment(x=w13) -> (x+1=w31:u64)
      n22 = Get Date/Time In Seconds() -> (seconds since 1Jan1904=w54:timestamp)
      n23 = To Double Precision Float(number=w54) -> (double precision float=w51:dbl)
      n24 = Increment(x=w31) -> (x+1=w27:u64)
      n25 = case shown="True" w16 {
        tunnel: w30 -> [_ w65]
        tunnel: w29 -> [_ w64]
        tunnel: w27 -> [_ w63]
        tunnel: [_ w62] -> w26
        tunnel: w17 -> [_ w61]
        frame False {
        }
        frame True {
          w67 = u64 1  # Uploaded
          w68 = u64 0  # idUser
          n26 = Get Date/Time In Seconds() -> (seconds since 1Jan1904=w69:timestamp)
          n27 = To Double Precision Float(number=w69) -> (double precision float=w66:dbl)
          n28 = Add(x=w61, y=99) -> (x+y=w71:i32)
          n29 = Increment(x=w63) -> (x+1=w72:u64)
          n30 = Bundle(w72, "idUser"=w68, w71, w66, "cRIO System Settings Cluster IN 2"=w65, "Administrator Cluster.Description"=w64, "Uploaded"=w67) -> (w62:T18)  [unwired: 1 in]
        }
      }
      n31 = Bundle(w31, "idUser"=w53, "tSetting_TypeDef"=tsettings_Core."Pan Cluster", w51, "Pan Cluster DEFAULT"=w45, "Administrator Cluster.Description"=w29, "Uploaded"=w52) -> (w47:T19)  [unwired: 1 in]
      n32 = Bundle(w27, "idUser"=w28, w38, w42, "cRIO System Settings Cluster IN"=w34, "Administrator Cluster.Description"=w29, "Uploaded"=w41) -> (w35:T20)  [unwired: 1 in]
      n33 = call <vilib>:"DB Tools Insert Data.vi"("data"=w47, "error in (no error)"=w48, "table"="tsettings", "connection reference"=w49) -> ("error out"=w36:errorcluster, "connection reference out"=w37:T16)  [unwired: 6 in]
      n34 = disable-structure shown="Enabled" {
        disable-tunnel: w37 -> [w90 w100]
        disable-tunnel: w36 -> [w89 w99]
        disable-tunnel: w35 -> [w87 _]
        disable-tunnel: [w84 w100] -> w32
        disable-tunnel: w26 -> [w83 _]
        disable-tunnel: [w82 w99] -> w25
        disable-tunnel: w16 -> [w81 _]
        frame Enabled {
          n35 = call <vilib>:"DB Tools Insert Data.vi"("data"=w87, "error in (no error)"=w89, "table"="tsettings", "connection reference"=w90) -> ("error out"=w85:errorcluster, "connection reference out"=w86:T16)  [unwired: 6 in]
          n36 = case shown="True" w81 {
            tunnel: w86 -> [w92 w97]
            tunnel: w85 -> [w91 w96]
            tunnel: [w92 w95] -> w84
            tunnel: w83 -> [_ w94]
            tunnel: [w91 w93] -> w82
            frame False {
            }
            frame True {
              n37 = call <vilib>:"DB Tools Insert Data.vi"("data"=w94, "error in (no error)"=w96, "table"="tsettings", "connection reference"=w97) -> ("error out"=w93:errorcluster, "connection reference out"=w95:T16)  [unwired: 6 in]
            }
          }
        }
        frame Disabled {
        }
      }
      n38 = call <vilib>:"DB Tools Close Connection.vi"("error in (no error)"=w25, "connection reference"=w32) -> ("error out"=→"error out":errorcluster)  [unwired: 5 in]
    }
    frame Disabled {
    }
  }
